vi "Cache User Parameters_new method.vi"(8 "error in (no error)":errorcluster, 11 "SHIFTER DATA in":T1) -> (0 "error out":errorcluster, 3 "SHIFTER DATA out":T1)   [LabVIEW 2013, in "main.lvlib"]
uses:
  main.lvlib
  Components/TypeDef - SHIFTER.ctl
  Components/Dependencies.llb/Exit Event Ref.ctl
  Controls/Reference Cluster.ctl
  Controls/Enum Variables.ctl
  Components/Dependencies.llb/TLB_Dependencies.lvlib
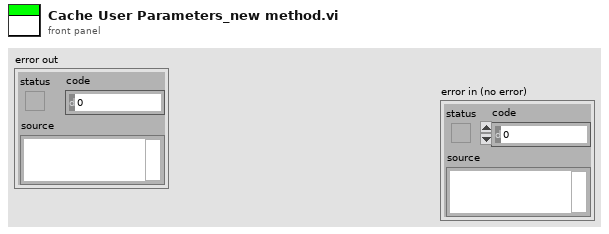
[diagram p1: front panel]
types:
  T1 = typedef "main.lvlib/TypeDef - SHIFTER.ctl" = cluster{"Exit Event":T2, "Terminate Error":errorcluster, "User Parameter Controls":refnum<vi>[], "User Parameters":cluster{"Name":string, "CPR Number":string, "Measuring Type ":string, "Measuring Technique":string, "Measuring Limb":string, "Operator":string, "Doctor":string, "Comment":string, "AdditionalInfo":string, "RightArm":string[][], "LeftArm":string[][], "PalpationRight":string, "PalpationLeft":string, "Puls":dbl, "Temp One":dbl, "Temp Two":dbl, "ActivityBox":bool}, "System Parameters":cluster{"Paper Running?":bool, "GraphSelection":bool, "Date":string, "Active Page":string}, "Data Acquisition":cluster{"Acquisition":bool, "DAQmx Task":refnum<k21>, "DAQmx Error":errorcluster, "Record number":dbl, "RecordPath":path, "AcqDataRef":refnum<vi>, "Duration":timestamp, "Queue":refnum<queue>, "Control?":bool, "RelativeRecordPath":path}, "Reference signal":cluster{"DAQmx  Task ":refnum<k21>, "Monitor":bool, "Events":dbl, "Time":timestamp, "NullEvents":dbl, "RefDataRef":refnum<vi>, "Queue":refnum<queue>}, "Data Process":cluster{"SubpanelRef":refnum<vi>, "ActiveItemTag":string, "Queue":refnum<queue>}, "System Parameter Controls":refnum<vi>[], "Database":cluster{"PatientdataRef":refnum<file>, "PatientdataPath":path, "Blue Pressure":dbl, "Red Pressure":dbl, "ActiveItemTag":string, "Height Adjustment":dbl, "BluePositionArray":dbl[][], "RedPositionArray":dbl[][], "JournalPath":path}, "MWL":cluster{"PatientID":string, "Name":string, "DICOM Info":path, "DICOM Variables":string[], "Worklist":string[][]}, "Control":cluster{"Queue":refnum<queue>, "SignalCluster":cluster{"Pump":bool, "Finger":bool, "Ankle":bool, "Fast Def":bool, "Slow Def":bool, "Init Cal":bool, "Table Pres":bool, "Table":bool}}, "PageMenu":cluster{"VI Reference":refnum<vi>, "Queue":refnum<queue>}, "Profile":cluster{"VI Reference":refnum<vi>, "Queue":refnum<queue>}, "Configuration":cluster{"VI Reference":refnum<vi>, "Queue":refnum<queue>}, "Acquisition":cluster{"VI Reference":refnum<vi>, "Queue":refnum<queue>}, "Data":cluster{"VI Reference":refnum<vi>, "Queue":refnum<queue>}, "Journal":cluster{"VI Reference":refnum<vi>, "Queue":refnum<queue>}, "cRef":T3, "Bluetooth":cluster{"Queue":refnum<queue>, "VI Reference":refnum<vi>}}
  T2 = typedef "main.lvlib/TLB_Dependencies.lvlib/Exit Event Ref.ctl" = refnum<user-event>
  T3 = typedef "main.lvlib/Reference Cluster.ctl" = cluster{"Menu":cluster{"References":cluster{"Stop Acq":refnum<vi>, "MenuExit":refnum<vi>, "MenuStartADC":refnum<vi>, "PersonalInfoString":refnum<vi>, "Profile":refnum<vi>, "Configuration":refnum<vi>, "Acquisition":refnum<vi>, "Data":refnum<vi>, "Journal":refnum<vi>}}, "Profile":cluster{"References":cluster{"Search Patient ID":refnum<vi>, "Name":refnum<vi>, "CommentStr":refnum<vi>, "Listbox Patient ID":refnum<vi>, "ListboxDoctor":refnum<vi>, "ListboxOperator":refnum<vi>, "HospitalName":refnum<vi>, "HospitalDepartment":refnum<vi>, "HospitalAddress":refnum<vi>, "EditHospInfo":refnum<vi>, "Add Patient ID Btn":refnum<vi>, "Query Worklist":refnum<vi>}}, "Configuration":cluster{"References":cluster{"ListboxMeasurementArea":refnum<vi>, "ListboxMeasurementTechnique":refnum<vi>, "ListboxMeasurementMeth":refnum<vi>, "ListboxRightSegmentNr":refnum<vi>, "ListboxLeftSegmentNr":refnum<vi>, "HeightAdjustmentInt":refnum<vi>, "PalpationRight":refnum<vi>, "PalpationLeft":refnum<vi>, "ActivityBox":refnum<vi>}, "New method":cluster{"AddNewMeasurementBtn":refnum<vi>, "Left Time Table":refnum<vi>, "Right Time Table":refnum<vi>}, "Old method":cluster{"LeftArmPressureTable":refnum<vi>, "RightArmPressureTable":refnum<vi>, "SaveArmPressureBtn":refnum<vi>, "Puls":refnum<vi>, "TempTwo":refnum<vi>, "TempOne":refnum<vi>}, "Method":string}, "Acquisition":cluster{"References":cluster{"SegmentAcqString":refnum<vi>, "RingActGraph":refnum<vi>}}, "Data":cluster{"References":cluster{"cmString":refnum<vi>, "AdjustedHeight":refnum<vi>, "Menu":refnum<vi>, "Tangent On/Off":refnum<vi>, "FilterControl":refnum<vi>}}, "Journal":cluster{"References":cluster{"ReportSelection":refnum<vi>, "Data":refnum<vi>, "GenerateReport":refnum<vi>, "Menu":refnum<vi>, "Send To PACS":refnum<vi>}}}
  T4 = typedef "main.lvlib/Enum Variables.ctl" = enum16{"SetAcqFilter", "GetAcqFilter", "Set Filter", "Get Filter", "Set Height", "Get Height", "Set Recorded Height", "Get Recorded Height", "Set Blue Pressure", "Get Blue Pressure", "Set Red Pressure", "Get Red Pressure", "Init", "Reset Pressure", "Set Red Cursors", "Get Red Cursors", "Set Blue Cursors", "Get Blue Cursors", "Set Language", "Get Language", "Set Active Graphs", "Get ActiveGraphs", "Set Method", "Get Method", "Set Encryption", "Get Encryption", "Set ExcelVersion", "Get ExcelVersion", "Set DICOM Avail", "Get DICOM Avail", "Set DICOM Encode", "Get DICOM Encode", "Set JournalExport", "Get JournalExport", "Set Sequence", "Get Sequence", "Set DAQ Connected", "Get DAQ Connected", "Set Current Graph", "Get Current Graph", "Set General Settings", "Get Hyphenation", "Set Arm Calc Method", "Get Arm Calc Method", "Set Dicom Tags", "Get Dicom Tags", "Set BT Serial", "Get BT Serial", "Set BT Accepted Serials", "Get BT Accepted Serials", "Get BT License", "Set BT License"}
  T5 = cluster{"Search Patient ID":refnum<vi>, "Name":refnum<vi>, "CommentStr":refnum<vi>, "Listbox Patient ID":refnum<vi>, "ListboxDoctor":refnum<vi>, "ListboxOperator":refnum<vi>, "HospitalName":refnum<vi>, "HospitalDepartment":refnum<vi>, "HospitalAddress":refnum<vi>, "EditHospInfo":refnum<vi>, "Add Patient ID Btn":refnum<vi>, "Query Worklist":refnum<vi>}
  T6 = cluster{"ListboxMeasurementArea":refnum<vi>, "ListboxMeasurementTechnique":refnum<vi>, "ListboxMeasurementMeth":refnum<vi>, "ListboxRightSegmentNr":refnum<vi>, "ListboxLeftSegmentNr":refnum<vi>, "HeightAdjustmentInt":refnum<vi>, "PalpationRight":refnum<vi>, "PalpationLeft":refnum<vi>, "ActivityBox":refnum<vi>}
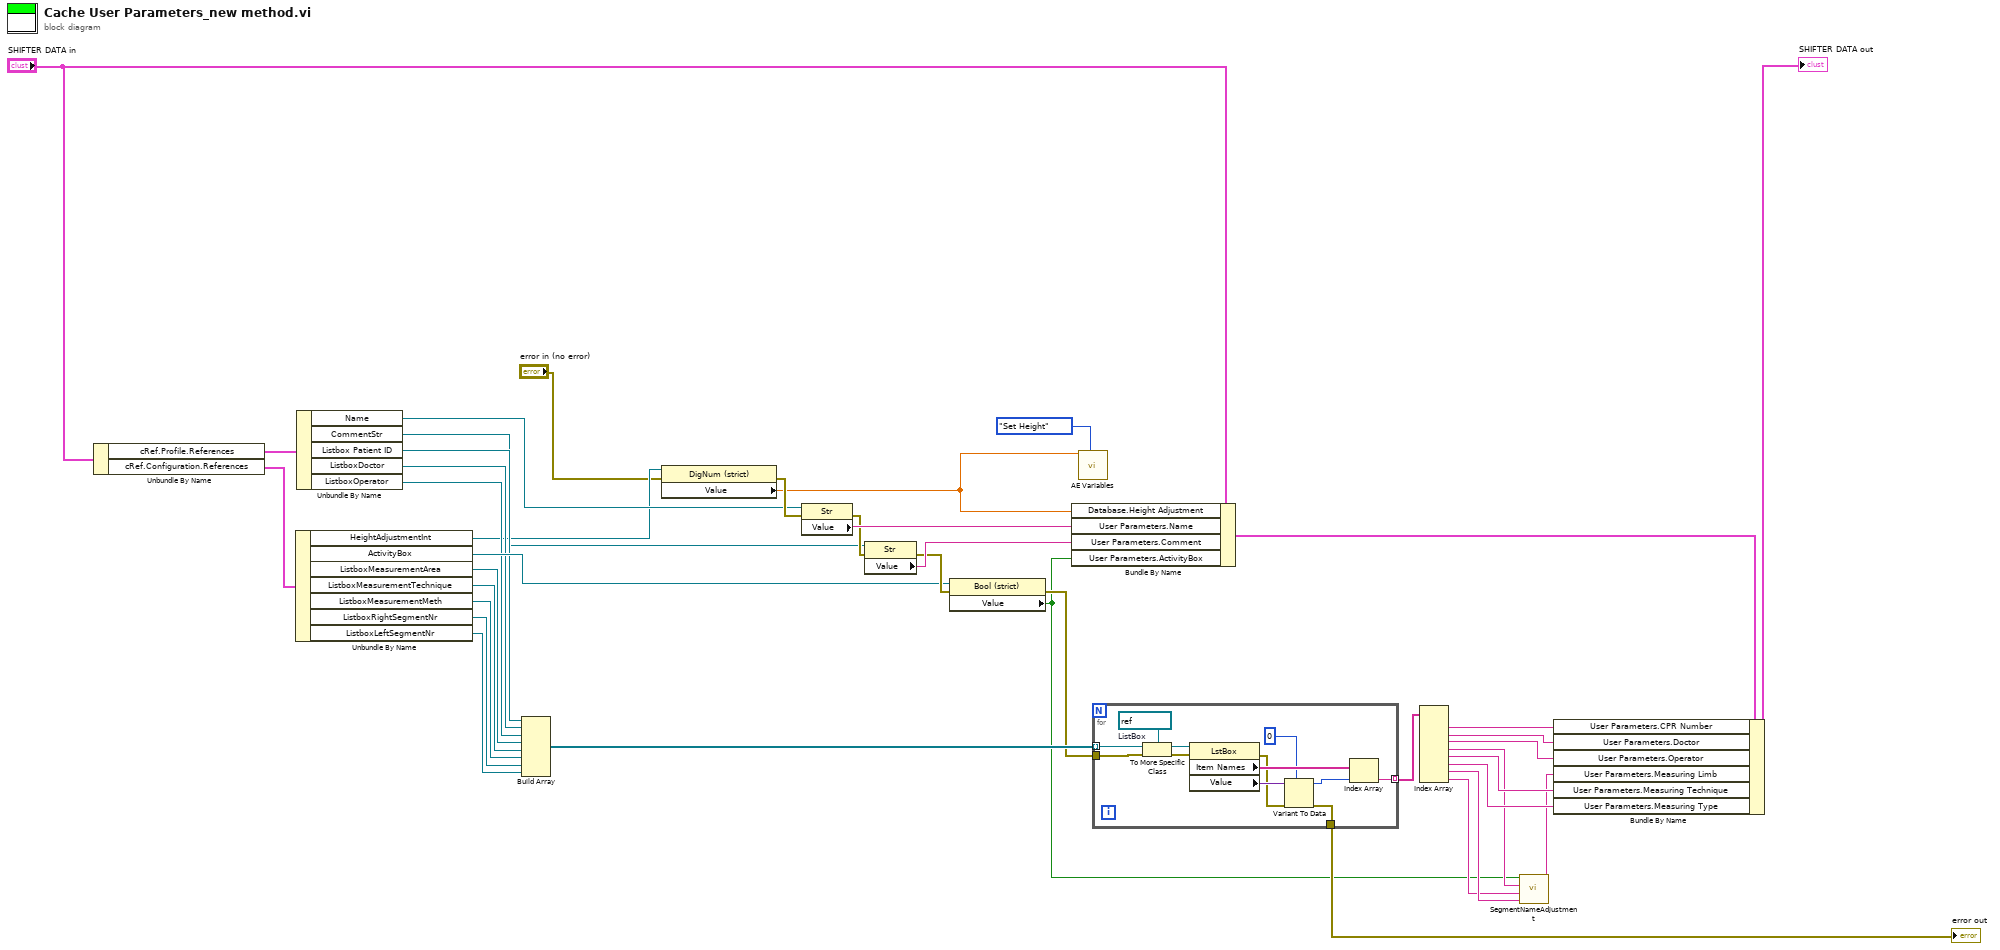
[diagram p0: block diagram]
diagram:
  n1 = Unbundle By Name("SHIFTER DATA in") -> ("cRef.Profile.References"=w11:T5, "cRef.Configuration.References"=w5:T6)
  n2 = Unbundle By Name(w5) -> ("HeightAdjustmentInt"=w4:refnum<vi>, "ActivityBox"=w12:refnum<vi>, "ListboxMeasurementArea"=w17:refnum<vi>, "ListboxMeasurementTechnique"=w16:refnum<vi>, "ListboxMeasurementMeth"=w15:refnum<vi>, "ListboxRightSegmentNr"=w14:refnum<vi>, "ListboxLeftSegmentNr"=w13:refnum<vi>)
  n3 = Unbundle By Name(w11) -> ("Name"=w6:refnum<vi>, "CommentStr"=w7:refnum<vi>, "Listbox Patient ID"=w8:refnum<vi>, "ListboxDoctor"=w9:refnum<vi>, "ListboxOperator"=w10:refnum<vi>)
  n4 = Build Array(w8, w9, w10, w17, w16, w15, w14, w13) -> (w34:refnum<vi>[])
  n5 = property class="DigNum (strict)"(reference=w4, error in="error in (no error)") -> (error out=w22:errorcluster, "Value"=w1:dbl)  [unwired: 1 out]
  n6 = property class="Str"(reference=w6, error in=w22) -> (error out=w21:errorcluster, "Value"=w23:string)  [unwired: 1 out]
  n7 = property class="Str"(reference=w7, error in=w21) -> (error out=w20:errorcluster, "Value"=w24:string)  [unwired: 1 out]
  n8 = property class="Bool (strict)"(reference=w12, error in=w20) -> (error out=w19:errorcluster, "Value"=w18:bool)  [unwired: 1 out]
  n9 = Bundle By Name(cluster="SHIFTER DATA in", "Database.Height Adjustment"=w1, "User Parameters.Name"=w23, "User Parameters.Comment"=w24, "User Parameters.ActivityBox"=w18) -> (w27:T1)
  n10 = call "AE Variables.vi"("VariantIn"=w1, "Action"=Enum_Variables."Set Height") -> ()  [unwired: 10 in, 8 out]
  n11 = for {
    tunnel: [w50] -> w35 mode=indexing
    tunnel: w34 -> [w49] mode=indexing
    tunnel: [w40] -> w39
    tunnel: w19 -> [w46]
    w48 = refnum<vi> refnum  # ListBox
    n12 = To More Specific Class(target class=w48, reference=w49, error in=w46) -> (specific class reference=w47:refnum<vi>, error out=w45:errorcluster)
    n13 = property class="LstBox"(reference=w47, error in=w45) -> (error out=w41:errorcluster, "Item Names"=w51:string[], "Value"=w44:variant)  [unwired: 1 out]
    n14 = Variant To Data(error in=w41, type=0, Variant=w44) -> (data=w42:i32, error out=w40:errorcluster)
    n15 = Index Array(array=w51, index=w42) -> (element=w50:string)
  }
  "error out" <- w39
  n16 = Index Array(array=w35) -> (element #1=w36:string, element #2=w26:string, element #3=w25:string, element #4=w32:string, element #5=w37:string, element #6=w38:string, element #7=w31:string, element #8=w30:string)  [unwired: 8 in]
  n17 = call "SegmentNameAdjustment.vi"("Right"=w31, "Left"=w30, "Segment In"=w32, "Activity"=w18) -> ("Segment Out"=w29:string)  [unwired: 7 in]
  n18 = Bundle By Name(cluster=w27, "User Parameters.CPR Number"=w36, "User Parameters.Doctor"=w26, "User Parameters.Operator"=w25, "User Parameters.Measuring Limb"=w29, "User Parameters.Measuring Technique"=w37, "User Parameters.Measuring Type"=w38) -> (→"SHIFTER DATA out":T1)
